vi "Draw Joystick.vi"(9 "Size":cluster{"X":u32, "Y":u32}, 11 "Mouse":T1) -> (1 "JS Coords":cluster{"X":dbl, "Y":dbl}, 3 "Arcade Inputs":picture)   [LabVIEW 2023]
uses:
  <vilib>/Utility/miscctls.llb/LVMouseTypeDef.ctl
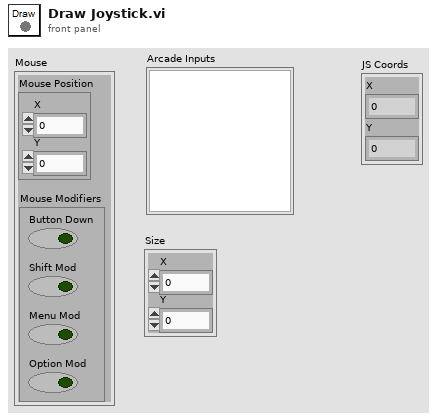
[diagram p1: front panel]
types:
  T1 = typedef "LVMouseTypeDef.ctl" = cluster{"Mouse Position":cluster{"X":i32, "Y":i32}, "Mouse Modifiers":cluster{"Button Down":bool, "Shift Mod":bool, "Menu Mod":bool, "Option Mod":bool}}
  T2 = cluster{"Button Down":bool, "Shift Mod":bool, "Menu Mod":bool, "Option Mod":bool}
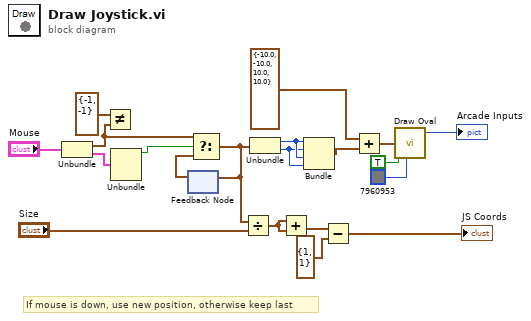
[diagram p0: block diagram]
diagram:
  # "If mouse is down, use new position, otherwise keep last"
  n1 = Unbundle("Mouse") -> ("Mouse Position"=w5:cluster{"X":i32, "Y":i32}, "Mouse Modifiers"=w4:T2)
  n2 = Not Equal?(x=cluster{"X":i32, "Y":i32} {"X"=-1, "Y"=-1}, y=w5) -> ()  [unwired: 1 out]
  n3 = Unbundle(w4) -> ("Button Down"=w3:bool)  [unwired: 3 out]
  n4 = feedback #1() -> (w1:cluster{"X":i32, "Y":i32})  [unwired: 1 in]
  n5 = Select(t=w5, s=w3, f=w1) -> (s? t:f=w2:cluster{"X":i32, "Y":i32})
  n6 = feedback-in #1(w2) -> ()
  n7 = Divide(x=w2, y="Size") -> (x/y=w9:cluster{"X":dbl, "Y":dbl})
  n8 = Unbundle(w2) -> ("X"=w16:i32, "Y"=w15:i32)
  n9 = Add(x=w9, y=w9) -> (x+y=w8:cluster{"X":dbl, "Y":dbl})
  n10 = Bundle("X"=w16, "Y"=w15, "X"=w16, "Y"=w15) -> (w14:cluster{"X":i32, "Y":i32, "X":i32, "Y":i32})  [unwired: 1 in]
  n11 = Subtract(x=w8, y=cluster{"X":i32, "Y":i32} {"X"=1, "Y"=1} ("x")) -> (x-y=→"JS Coords":cluster{"X":dbl, "Y":dbl})
  n12 = Add(x=cluster{"X":dbl, "Y":dbl, "X":dbl, "Y":dbl} {"X"=-10.0, "Y"=-10.0, "X"=10.0, "Y"=10.0}, y=w14) -> (x+y=w12:cluster{"X":dbl, "Y":dbl, "X":dbl, "Y":dbl})
  n13 = call <vilib>:"Draw Oval.vi"("rect"=w12, "fill?(F)"=TRUE, "color(black)"=u32 7960953) -> ("new picture"=→"Arcade Inputs":picture)  [unwired: 6 in]
